vi "New GUID.vi"() -> (3 "ToString":string)   [LabVIEW 2019, in "Redis Client Examples.lvlib"]
uses:
  Redis Client Examples.lvlib
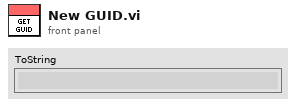
[diagram p1: front panel]
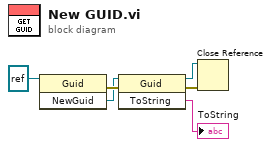
[diagram p0: block diagram]
diagram:
  n1 = invoke class="Guid" method="NewGuid"(reference=refnum<k24> refnum) -> (error out=w3:errorcluster, "NewGuid"=w1:refnum<k24>)  [unwired: 2 in, 1 out]
  n2 = invoke class="Guid" method="ToString"(reference=w1, error in=w3) -> (reference out=w5:refnum<k24>, error out=w4:errorcluster, "ToString"=→"ToString":string)  [unwired: 1 in]
  n3 = Close Reference(reference=w5, error in (no error)=w4) -> ()  [unwired: 1 out]
